vi "PWM.vi"(2 "Force time?":bool, 3 "Forced Time":dbl, 4 "Reset":bool, 5 "Initialize?":bool, 6 "On Period":dbl, 7 "Total Period":dbl) -> (0 "OUTPUT":bool, 1 "Time":dbl)   [LabVIEW 2021]
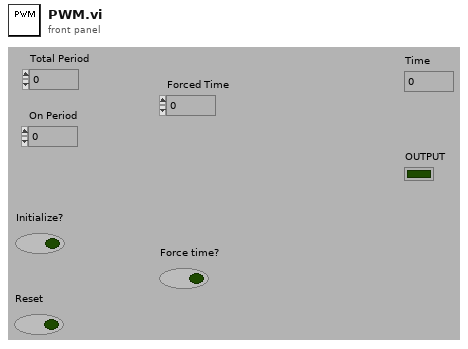
[diagram p1: front panel]
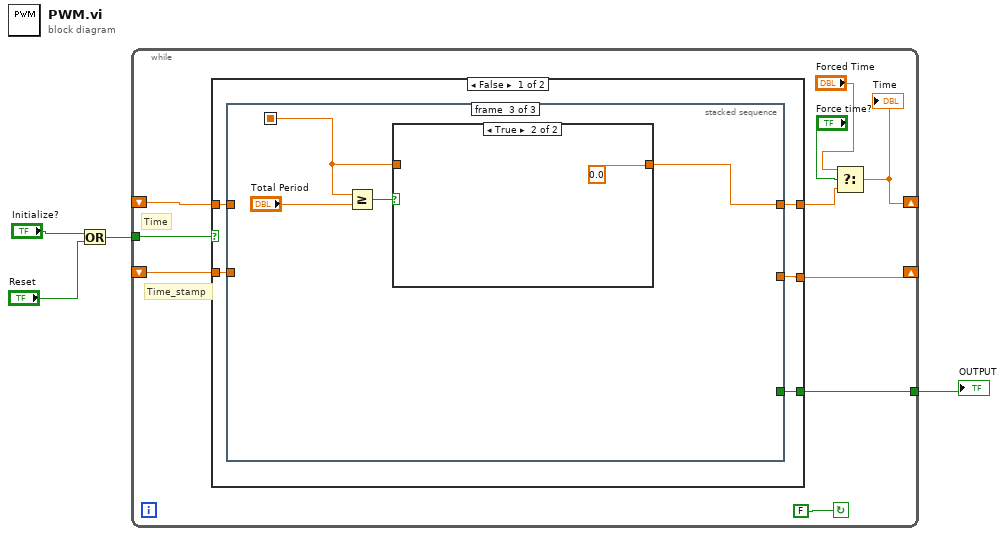
[diagram p0: block diagram]
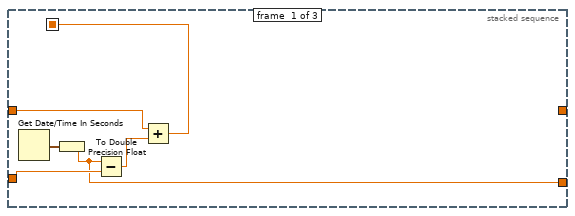
[diagram p2: hidden frame]
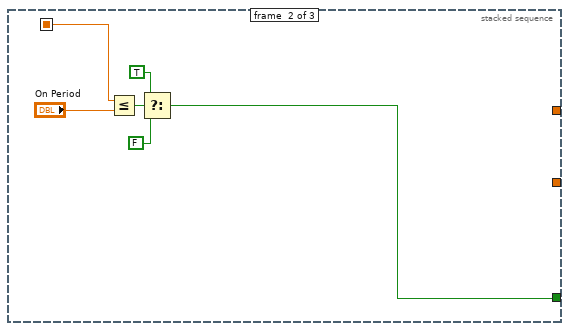
[diagram p3: hidden frame]
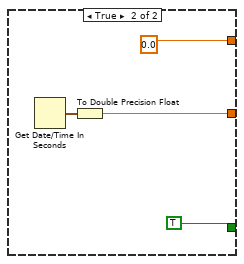
[diagram p5: hidden frame]
diagram:
  n1 = Or(x="Initialize?", y="Reset") -> (x .or. y?=w4:bool)
  n2 = while {
    shift-right: [w6] -> _
    shift-left: _ -> [w9]
    shift-right: [w11] -> _
    shift-left: _ -> [w12]
    tunnel: w4 -> [w13]
    tunnel: [w10] -> w1
    stop <- FALSE continue-if-true
    # "Time_stamp"
    # "Time"
    n3 = case shown="False" w13 {
      tunnel: w9 -> [w18 _]
      tunnel: w12 -> [w19 _]
      tunnel: [w17 w40] -> w11
      tunnel: [w16 0.0] -> w7
      tunnel: [w15 TRUE] -> w10
      frame False {
        n4 = stacked-sequence {
          seq-local: [w20 _ _] -> [_ w30 w33]
          tunnel: w19 -> [w24 _ _]
          tunnel: w18 -> [w22 _ _]
          tunnel: [w21 _ _] -> w17
          tunnel: [_ _ w32] -> w16
          tunnel: [_ w26 _] -> w15
          frame #0 {
            n5 = Get Date/Time In Seconds() -> (seconds since 1Jan1904=w25:timestamp)
            n6 = To Double Precision Float(number=w25) -> (double precision float=w21:dbl)
            n7 = Subtract(x=w21, y=w24) -> (x-y=w23:dbl)
            n8 = Add(x=w22, y=w23) -> (x+y=w20:dbl)
          }
          frame #1 {
            n9 = Less Or Equal?(x=w30, y="On Period") -> (x <= y?=w31:bool)
            n10 = Select(t=TRUE, s=w31, f=FALSE) -> (s? t:f=w26:bool)
          }
          frame #2 {
            n11 = Greater Or Equal?(x=w33, y="Total Period") -> (x >= y?=w34:bool)
            n12 = case shown="True" w34 {
              tunnel: w33 -> [w36 _]
              tunnel: [w36 0.0] -> w32
              frame False {
              }
              frame True {
              }
            }
          }
        }
      }
      frame True {
        n13 = Get Date/Time In Seconds() -> (seconds since 1Jan1904=w41:timestamp)
        n14 = To Double Precision Float(number=w41) -> (double precision float=w40:dbl)
      }
    }
    n15 = Select(t="Forced Time", s="Force time?", f=w7) -> (s? t:f=w6:dbl)
    "Time" <- w6
  }
  "OUTPUT" <- w1
